vi "CurveFinished Event Callback.vi"(4 "User Parameter":T2, 5 "Event Data":cluster{"sender":refnum<k24>, "e":refnum<k24>}, 6 "Control Ref":refnum<k24>, 7 "Event Common Data":T3) -> ()   [LabVIEW 2025]
uses:
  C:/Users/stef/code/palmsenssdk/labview/PalmSens/Libraries/PalmSens.Core.Simplified.LabVIEW.dll
  Libraries/PalmSens.Core.Simplified.LabVIEW.dll
  ActiveCurve.ctl
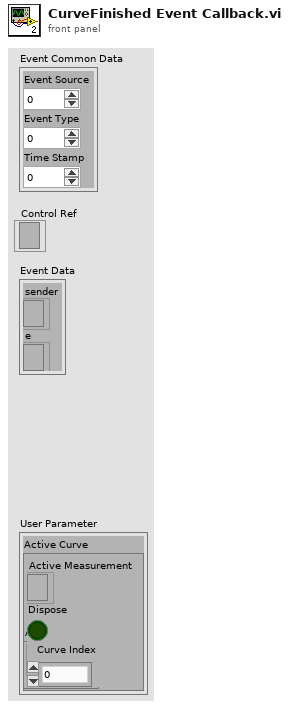
[diagram p1: front panel]
types:
  T1 = typedef "ActiveCurve.ctl" = cluster{"Active Measurement":refnum<k24>, "Dispose":bool, "Curve Index":i32}
  T2 = cluster{"Active Curve":T1, "Active Curve Event":refnum<user-event>}
  T3 = cluster{"Event Source":i32, "Event Type":u32, "Time Stamp":u32}
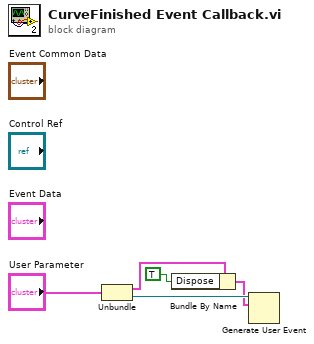
[diagram p0: block diagram]
diagram:
  n1 = Unbundle("User Parameter") -> ("Active Curve"=w3:T1, "Active Curve Event"=w4:refnum<user-event>)
  n2 = Bundle By Name(cluster=w3, "Dispose"=TRUE) -> (w1:T1)
  n3 = Generate User Event(user event=w4, event data cluster=w1) -> ()  [unwired: 2 in, 2 out]
